vi "OceanExample.vi"() -> ()   [LabVIEW 2022 SP3]
uses:
  C:/Program Files (x86)/Ocean Optics/OmniDriverSPAM/OOI_HOME/NETOmniDriver-NET40.dll
panel:
  out "isSaturated":bool
  out "isSpectrumValid":bool
  out "Spectrometer Name:":string
  out "Serial Number:":string
  in  "Scans to Average":i32=1 min=1 max=50 step=1
  in  "Boxcar Width":i32 min=0 max=50 step=1
  in  "Int. Time (microsec)":i32=10000 min=10000
  out "Number of Spectrometers":i32
  in  "stop":bool
  out "Current Spectrum":cluster{"Y":dbl[], "Y":dbl[]}[](graph)
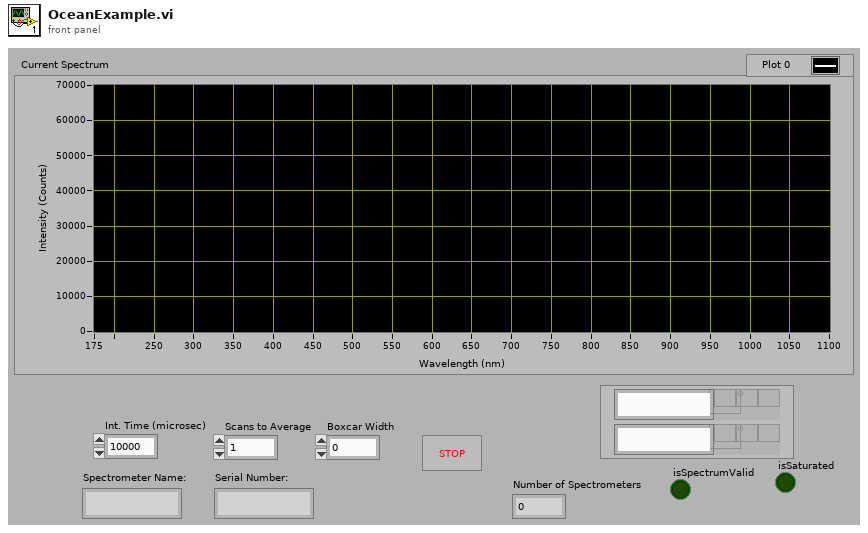
[diagram p1: front panel]
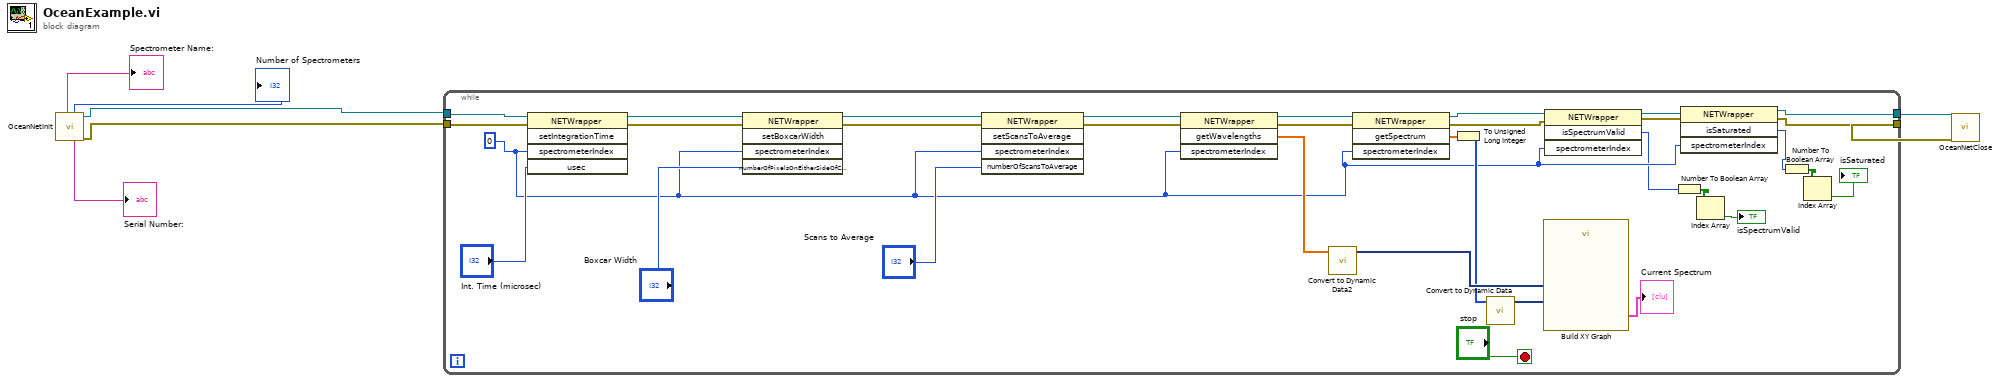
[diagram p0: block diagram]
diagram:
  n1 = call "OceanNetInit.vi"() -> ("error out"=w5:errorcluster, "Ocean. NET out"=w2:refnum<k24>, "Serial Number:"=→"Serial Number:":string, "Number of Spectrometers"=→"Number of Spectrometers":i32, "Spectrometer Name:"=→"Spectrometer Name:":string)  [unwired: 6 in, 1 out]
  n2 = while {
    tunnel: [w17] -> w7
    tunnel: [w18] -> w6
    tunnel: w2 -> [w34]
    tunnel: w5 -> [w33]
    stop <- "stop" stop-if-true
    w14 = 0
    n3 = invoke class="NETWrapper" method="setIntegrationTime"(reference=w34, error in=w33, "spectrometerIndex"=w14, "usec"="Int. Time (microsec)") -> (reference out=w30:refnum<k24>, error out=w29:errorcluster)  [unwired: 1 in, 3 out]
    n4 = invoke class="NETWrapper" method="setBoxcarWidth"(reference=w30, error in=w29, "spectrometerIndex"=w14, "numberOfPixelsOnEitherSideOfCenter"="Boxcar Width") -> (reference out=w28:refnum<k24>, error out=w27:errorcluster)  [unwired: 1 in, 3 out]
    n5 = invoke class="NETWrapper" method="setScansToAverage"(reference=w28, error in=w27, "spectrometerIndex"=w14, "numberOfScansToAverage"="Scans to Average") -> (reference out=w25:refnum<k24>, error out=w24:errorcluster)  [unwired: 1 in, 3 out]
    n6 = invoke class="NETWrapper" method="getWavelengths"(reference=w25, error in=w24, "spectrometerIndex"=w14) -> (reference out=w40:refnum<k24>, error out=w39:errorcluster, "getWavelengths"=w22:dbl[])  [unwired: 1 in, 1 out]
    n7 = call "Convert to Dynamic Data2"("Array"=w22) -> ("Dynamic Data Type"=w38:dynamicdata)  [unwired: 3 out]
    n8 = invoke class="NETWrapper" method="getSpectrum"(reference=w40, error in=w39, "spectrometerIndex"=w14) -> (reference out=w20:refnum<k24>, error out=w15:errorcluster, "getSpectrum"=w23:dbl[])  [unwired: 1 in, 1 out]
    n9 = To Unsigned Long Integer(number=w23) -> (unsigned 32bit integer=w21:u32[])
    n10 = call "Convert to Dynamic Data"("Array"=w21) -> ("Dynamic Data Type"=w37:dynamicdata)  [unwired: 3 out]
    n11 = call "Build XY Graph"("Y Input"=w37, "X Input"=w38) -> ("XY Graph"=→"Current Spectrum":cluster{"Y":dbl[], "Y":dbl[]}[])  [unwired: 3 in, 6 out]
    n12 = invoke class="NETWrapper" method="isSpectrumValid"(reference=w20, error in=w15, "spectrometerIndex"=w14) -> (reference out=w19:refnum<k24>, error out=w16:errorcluster, "isSpectrumValid"=w13:i16)  [unwired: 1 in, 1 out]
    n13 = Number To Boolean Array(number=w13) -> (Boolean array=w12:bool[])
    n14 = invoke class="NETWrapper" method="isSaturated"(reference=w19, error in=w16, "spectrometerIndex"=w14) -> (reference out=w18:refnum<k24>, error out=w17:errorcluster, "isSaturated"=w10:i16)  [unwired: 1 in, 1 out]
    n15 = Index Array(array=w12) -> (element=→"isSpectrumValid":bool)  [unwired: 1 in]
    n16 = Number To Boolean Array(number=w10) -> (Boolean array=w9:bool[])
    n17 = Index Array(array=w9) -> (element=→"isSaturated":bool)  [unwired: 1 in]
  }
  n18 = call "OceanNetClose.vi"("error in (no error)"=w7, ".NET Refnum in"=w6) -> ()  [unwired: 10 in]
